vi "Test Evaluate Part 2 attempt 2.vi"() -> ()   [LabVIEW 2020]
uses:
  Proto/Proto.lvclass
panel:
  out "x = y?":bool
  out "number":u64
  out "Array":bool[](array[boolean])
  in  "Input":string="x00: 1\nx01: 0\nx02: 1\nx03: 1\nx04: 0\ny00: 1\ny01: 1\ny02: 1\ny03: 1\ny04: 1\n\nntg XOR fgs -> mjb\ny02 OR x01 -> tnw\nkwq OR kpj -> z05\nx00 OR x03 -> fst\ntgd XOR rvg -> z01\nvdt OR tnw -> bfw\nbfw AND frj -> z10\nffh OR nrd -> bqk\ny00 AND y03 -> djm\ny03 OR y00 -> psh\nbqk OR frj -> z08\ntnw OR fst -> frj\ngnj AND tgd -> z11\nbfw XOR mjb -> z00\nx03 OR x00 -> vdt\ngnj AND wpb -> z02\nx04 AND y00 -> kjc\ndjm OR pbm -> qhw\nnrd AND vdt -> hwm\nkjc AND fst -> rvg\ny04 OR y02 -> fgs\ny01 AND x02 -> pbm\nntg OR kjc -> kwq\npsh XOR fgs -> tgd\nqhw XOR tgd -> z09\npbm OR djm -> kpj\nx03 XOR y03 -> ffh\nx00 XOR y04 -> ntg\nbfw OR bqk -> z06\nnrd XOR fgs -> wpb\nfrj XOR qhw -> z04\nbqk OR frj -> z07\ny03 OR x01 -> nrd\nhwm AND bqk -> z03\ntgd XOR rvg -> z12\ntnw OR pbm -> gnj"
  # "2947015374 too low\n\n282578783305985 too high\n66055249060558"
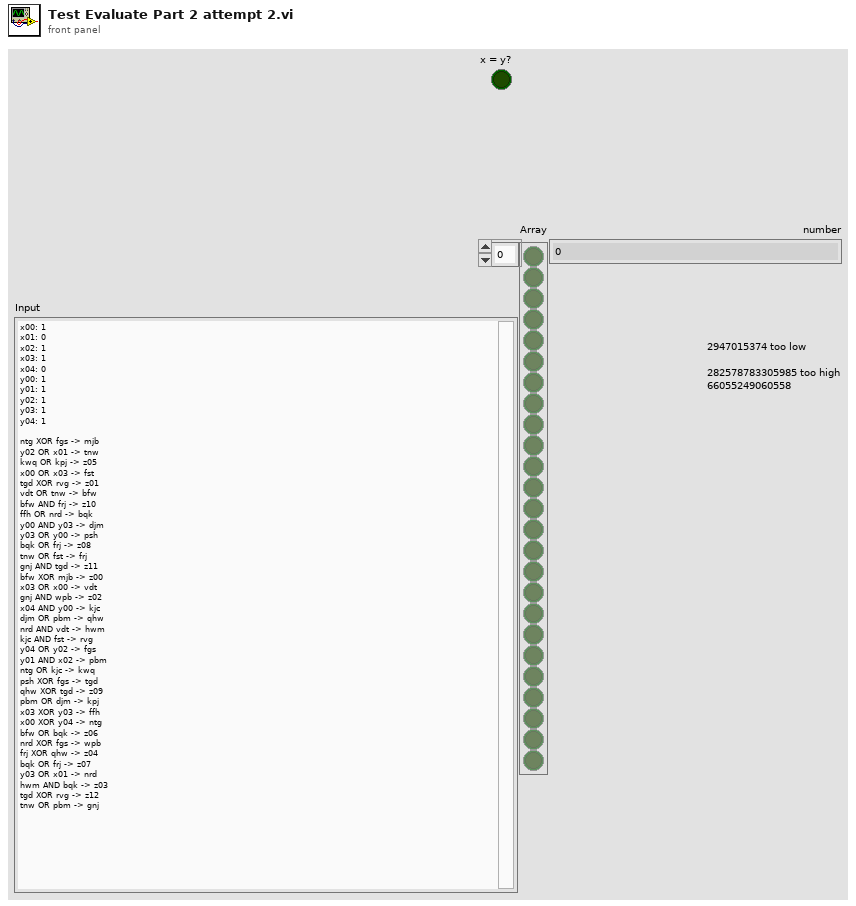
[diagram p1: front panel]
types:
  T1 = cluster{u64, cluster{"String":string, "String":string}}[]
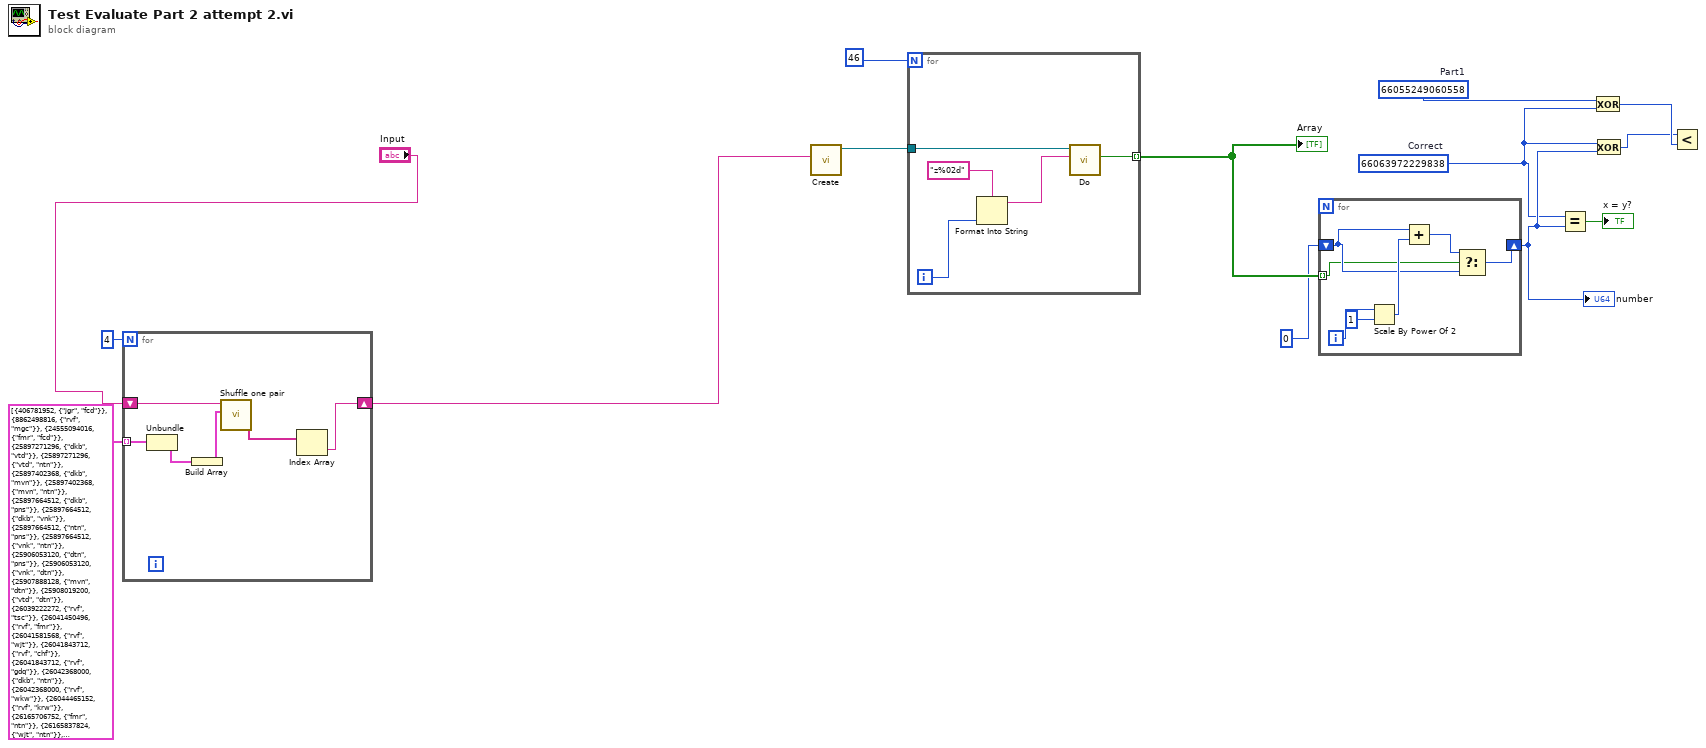
[diagram p0: block diagram]
diagram:
  w4 = u64 66055249060558  # Part1
  w3 = u64 66063972229838  # Correct
  n1 = for {
    N: 4 -> [_]
    tunnel: T1 [{406781952, {"String"="jgr", "String"="fcd"}}, {8862498816, {"String"="rvf", "String"="mgc"}}, {24555094016, {"String"="fmr", "String"="fcd"}}, {25897271296, {"String"="dkb", "String"="vtd"}}, {25897271296, {"String"="vtd", "String"="ntn"}}, {25897402368, {"String"="dkb", "String"="mvn"}}, {25897402368, {"String"="mvn", "String"="ntn"}}, {25897664512, {"String"="dkb", "String"="pns"}}, {25897664512, {"String"="dkb", "String"="vnk"}}, {25897664512, {"String"="ntn", "String"="pns"}}, {25897664512, {"String"="vnk", "String"="ntn"}}, {25906053120, {"String"="dtn", "String"="pns"}}, {25906053120, {"String"="vnk", "String"="dtn"}}, {25907888128, {"String"="mvn", "String"="dtn"}}, {25908019200, {"String"="vtd", "String"="dtn"}}, {26039222272, {"String"="rvf", "String"="tsc"}}, {26041450496, {"String"="rvf", "String"="fmr"}}, {26041581568, {"String"="rvf", "String"="wjt"}}, {26041843712, {"String"="rvf", "String"="chf"}}, {26041843712, {"String"="rvf", "String"="gdq"}}, {26042368000, {"String"="dkb", "String"="ntn"}}, {26042368000, {"String"="rvf", "String"="wkw"}}, {26044465152, {"String"="rvf", "String"="krw"}}, {26165706752, {"String"="fmr", "String"="ntn"}}, {26165837824, {"String"="wjt", "String"="ntn"}}, {26166099968, {"String"="chf", "String"="ntn"}}, {26166099968, {"String"="gdq", "String"="ntn"}}, {26166099968, {"String"="krw", "String"="ntn"}}, {26166099968, {"String"="ntn", "String"="tsc"}}, {26173046784, {"String"="vtd", "String"="tsc"}}, {26173177856, {"String"="mvn", "String"="tsc"}}, {26173571072, {"String"="fmr", "String"="pns"}}, {26173702144, {"String"="wjt", "String"="pns"}}, {26173964288, {"String"="chf", "String"="pns"}}, {26173964288, {"String"="gdq", "String"="pns"}}, {26174095360, {"String"="fmr", "String"="vnk"}}, {26174226432, {"String"="vnk", "String"="wjt"}}, {26174488576, {"String"="chf", "String"="vnk"}}, {26174488576, {"String"="gdq", "String"="vnk"}}, {26174488576, {"String"="vnk", "String"="tsc"}}, {26174488576, {"String"="vnk", "String"="wkw"}}, {26174488576, {"String"="wkw", "String"="pns"}}, {26175668224, {"String"="vtd", "String"="chf"}}, {26175668224, {"String"="vtd", "String"="wjt"}}, {26175799296, {"String"="chf", "String"="mvn"}}, {26175799296, {"String"="gdq", "String"="mvn"}}, {26175930368, {"String"="vtd", "String"="gdq"}}, {26176192512, {"String"="fmr", "String"="chf"}}, {26176192512, {"String"="fmr", "String"="tsc"}}, {26176192512, {"String"="vtd", "String"="vnk"}}, {26176323584, {"String"="chf", "String"="wjt"}}, {26176323584, {"String"="mvn", "String"="wkw"}}, {26176323584, {"String"="vnk", "String"="mvn"}}, {26176323584, {"String"="wjt", "String"="tsc"}}, {26176454656, {"String"="fmr", "String"="mvn"}}, {26176454656, {"String"="fmr", "String"="wjt"}}, {26176454656, {"String"="vtd", "String"="wkw"}}] ("sorted array") -> [w19] mode=indexing
    tunnel: [w19] -> _ mode=indexing
    shift-right: [w15] -> w11
    shift-left: "Input" -> [w20]
    n2 = Unbundle(w19) -> (w18:cluster{"String":string, "String":string})  [unwired: 1 out]
    n3 = Build Array(w18) -> (w17:cluster{"String":string, "String":string}[])
    n4 = call "Shuffle one pair.vi"("Array in"=w17, "Input"=w20) -> ("Array out"=w16:string[])  [unwired: 9 in]
    n5 = Index Array(array=w16) -> (element=w15:string)  [unwired: 1 in]
  }
  n6 = call "Create.vi"("Input"=w11) -> ("Proto"=w10:refnum<class "Proto.lvclass">)  [unwired: 9 in, 1 out]
  n7 = for {
    N: 46 -> [_]
    tunnel: w10 -> [w25]
    tunnel: [w21] -> w9 mode=indexing
    i -> [w23]
    n8 = Format Into String(format string="z%02d", w23) -> (resulting string=w22:string)  [unwired: 2 in, 1 out]
    n9 = call "Do.vi"("Key"=w22, "Proto in"=w25) -> ("Value"=w21:bool)  [unwired: 7 in, 2 out]
  }
  "Array" <- w9
  n10 = for {
    tunnel: w9 -> [w28] mode=indexing
    shift-right: [w26] -> w5
    shift-left: u64 0 ("number") -> [w29]
    i -> [w32]
    n11 = Scale By Power Of 2(n=w32, x=u64 1) -> (x*2^n=w30:u64)
    n12 = Add(x=w29, y=w30) -> (x+y=w27:u64)
    n13 = Select(t=w27, s=w28, f=w29) -> (s? t:f=w26:u64)
  }
  "number" <- w5
  n14 = Equal?(x=w3, y=w5) -> (x = y?=→"x = y?":bool)
  n15 = Exclusive Or(1:w3, 2:w4) -> (0:w2:u64)
  n16 = Exclusive Or(1:w5, 2:w3) -> (0:w1:u64)
  n17 = Less?(x=w1, y=w2) -> ()  [unwired: 1 out]
